vi "Write GridView Enqueuer.vi"(8 "error in (no error)":errorcluster, 10 "Actor Framework:Message Enqueuer":refnum<class "Message Enqueuer.lvclass">, 11 "DemoMain in":refnum<class "DemoMain.lvclass">) -> (0 "error out":errorcluster, 3 "DemoMain out":refnum<class "DemoMain.lvclass">)   [LabVIEW 2012, in "Win8uiDemo.lvlib" / "DemoMain.lvclass"]
uses:
  DemoMain.lvclass
  <vilib>/ActorFramework/Message Enqueuer/Message Enqueuer.lvclass
  DemoMain.lvclass/DemoMain.ctl
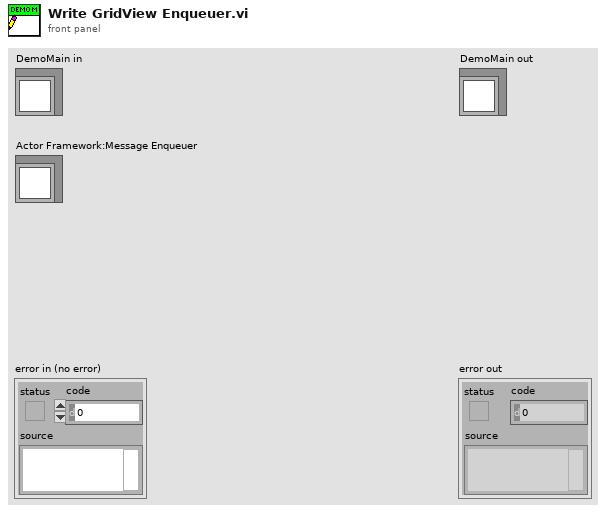
[diagram p1: front panel]
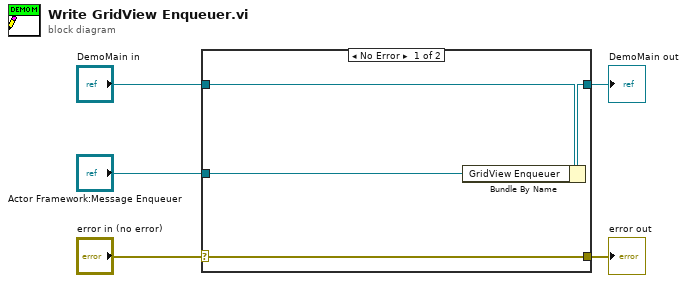
[diagram p0: block diagram]
diagram:
  n1 = case shown="No Error" "error in (no error)" {
    selector: "error in (no error)" -> [w9 w10]
    tunnel: [w9 w10] -> w4
    tunnel: [w7 w11] -> w2
    tunnel: "DemoMain in" -> [w8 w11]
    tunnel: "Actor Framework:Message Enqueuer" -> [w6 _]
    frame No Error {
      n2 = Bundle By Name(cluster=w8, "GridView Enqueuer"=w6) -> (w7:refnum<class "DemoMain.lvclass">)
    }
    frame Error {
    }
  }
  "error out" <- w4
  "DemoMain out" <- w2
